vi "strerror.vi"(11 "status_code":u32(ring) items=["APDM_OK"=0, "APDM_INVALID_PARAM"=1, "APDM_MISSED_DATA"=2, "APDM_INITIALIZATION_ERROR"=3, "APDM_NO_MORE_DATA"=4, "APDM_FT_COMMUNICATIONS_ERROR"=5, "APDM_STATUS_ERROR"=6, "APDM_STATUS_UNKNOWN"=7, "APDM_MEMORY_ALLOCATION_ERROR"=8, "APDM_INSUFFICIENT_RESOURCES"=9, "APDM_COMMUNICATIONS_ERROR"=10, "APDM_NOT_ENOUGH_ACCESS_POINTS"=11, "APDM_INVALID_FIRMWARE"=12, "APDM_CANT_RESET_INTO_TARGET_MODE"=13, "APDM_FIRMWARE"=14, "APDM_BOOTLOADER"=15, "APDM_INVALID_CONTEXT_HANDLE"=16, "APDM_CRC16_ERROR"=17, "APDM_DEVICE_RESPONSE_ERROR"=18, "APDM_DEVICE_FIRMWARE_TOO_OLD"=19, "APDM_FILE_ERROR"=20, "APDM_UNSUPPORTED_DEVICE_FIRMWARE_VERSION"=21, "APDM_UNSUPPORTED_DOCKING_STATION_FIRMWARE_VERSION"=22, "APDM_UNSUPPORTED_AP_FIRMWARE_VERSION"=23, "APDM_UNSUPPORTED_CALIBRATION_DATA_VERSION"=24, "APDM_SYNC_LINE_ERROR"=25, "APDM_UNKNOWN_SENSOR_ID_ERROR"=26, "APDM_DEVICE_NOT_FOUND"=27, "APDM_UNSUPPORTED_COMMAND"=28, "APDM_DEVICE_TX_RX_COLLISION_ERROR"=29, "APDM_READ_TIMEOUT_ERROR"=30, "APDM_UNABLE_TO_SYNC_RECORD_HEAD_LIST_ERROR"=31, "APDM_UNKNOWN_CALIBRATION_DATA_STRUCTURE"=32, "APDM_NULL_PARAMETER_ERROR"=33, "APDM_NOT_FOUND"=34, "APDM_UNKNOWN_DEVICE_TYPE"=35, "APDM_NO_CORRELATION_FIFO"=36, "APDM_UNSUPPORTED_DATA_FILE_VERSION"=37, "APDM_CORRUPT_DISK_FIFO"=38, "APDM_DOCK_UNSUPPORTED_HOST_LIBRARY_VERSION"=39, "APDM_AP_UNSUPPORTED_HOST_LIBRARY_VERSION"=40, "APDM_UNEXPECTED_STRUCTURE_VALUE"=41, "APDM_BAD_DATA"=42, "APDM_CORRUPT_CONTEXT"=43, "APDM_AP_READ_TIMEOUT_ERROR"=44, "APDM_MONITOR_READ_TIMEOUT_ERROR"=45, "APDM_DOCK_READ_TIMEOUT_ERROR"=46, "APDM_DEVICE_RESPONSE_ERROR_CRC_ERROR"=47, "APDM_DEVICE_RESPONSE_ERROR_INVALID_COMMAND"=48, "APDM_DEVICE_RESPONSE_ERROR_INVALID_PARAM_SIZE"=49, "APDM_DEVICE_RESPONSE_ERROR_INVALID_PARAM_VALUE"=50, "APDM_DEVICE_RESPONSE_ERROR_ERROR_EXECUTING_COMMAND"=51, "APDM_RECALIBRATION_INSUFFICIENT_DATA"=52, "APDM_RECALIBRATION_BAD_FIT"=53, "APDM_RECALIBRATION_INSUFFICIENT_MOVEMENT"=54, "APDM_FIRMWARE_COMBINATION_ERROR"=55, "APDM_DATA_FROM_UNEXPECTED_MONITOR_ERROR"=56, "APDM_ORIENTATION_ERROR"=57, "APDM_UNABLE_TO_PING_MONITOR_ERROR"=58, "APDM_FIRMWARE_INCOMPATABLE"=59, "APDM_INVALID_MONITOR_CONFIGURATION"=60, "APDM_UNABLE_TO_MATCH_EXPECTED_AP_IDS"=61, "APDM_AP_LIBUSB_ERROR_NO_DEVICE"=62, "APDM_DOCK_LIBUSB_ERROR_NO_DEVICE"=63, "APDM_UNSUPPORTED_AP_HANDLE_VERSION"=64, "APDM_NOT_V1_AP_HANDLE"=65, "APDM_NOT_V2_AP_HANDLE"=66, "APDM_NOT_V1_DOCK_HANDLE"=67, "APDM_NOT_V2_MONITOR_HANDLE"=68, "APDM_HANDLE_VERSION_UNKNOWN"=69, "APDM_CANT_MIX_HARDWARE_VERSIONS"=70, "APDM_CORRELATION_ERROR"=71, "APDM_NOT_ENOUGH_MONITORS"=72, "APDM_NO_FILE_OVERLAP"=73, "APDM_ECHO_SYNC_ERROR"=74, "APDM_AP_NOT_READY_TO_STREAM"=75, "APDM_INTERPOLATION_ERROR"=76, "APDM_ASYNC_MODE_RESPONSE"=77, "APDM_COMMUNICATION_MAGIC_NUMBER_ERROR"=78, "APDM_SENSOR_RESET_DURING_STREAMING"=79, "APDM_HDF_ERROR"=80, "APDM_BUFFER_VALIDATION"=81, "APDM_DECOMPRESSION_ERROR"=82, "APDM_DATA_COMM_CRC_ERROR"=83, "APDM_INCORRECT_NUMBER_OF_APS_CONNECTED"=84, "APDM_LIB_USB_ERROR"=2000, "APDM_LIBUSB_ERROR_IO"=2001, "APDM_LIBUSB_ERROR_INVALID_PARAM"=2002, "APDM_LIBUSB_ERROR_ACCESS"=2003, "APDM_LIBUSB_ERROR_NO_DEVICE"=2004, "APDM_LIBUSB_ERROR_NOT_FOUND"=2005, "APDM_LIBUSB_ERROR_BUSY"=2006, "APDM_LIBUSB_ERROR_TIMEOUT"=2007, "APDM_LIBUSB_ERROR_OVERFLOW"=2008, "APDM_LIBUSB_ERROR_PIPE"=2009, "APDM_LIBUSB_ERROR_INTERRUPTED"=2010, "APDM_LIBUSB_ERROR_NO_MEM"=2011, "APDM_LIBUSB_ERROR_NOT_SUPPORTED"=2012, "APDM_LIBUSB_ERROR_UNKOWN"=2098, "APDM_LIBUSB_ERROR_OTHER"=2099, "APDM_FTDI_COMM_ERROR"=3000]) -> (3 "function return":string)   [LabVIEW 2019, in "apdm.lvlib"]
doc: "APDM_EXPORT const char* apdm_strerror(const enum APDM_Status status_code);"
uses:
  apdm.lvlib
  Lee Lab/CP FES Walking 2018/Code/Working/LabVIEW/apdm.dll
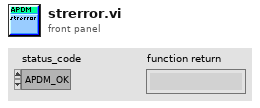
[diagram p1: front panel]
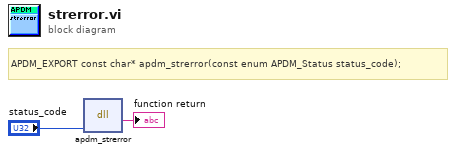
[diagram p0: block diagram]
diagram:
  # "APDM_EXPORT const char* apdm_strerror(const enum APDM_Status status_code);"
  n1 = dll-call lib="C:/Users/jfalesi/Dropbox/Lee Lab/CP FES Walking 2018/Code/Working/LabVIEW/apdm.*" fn="apdm_strerror"("status_code"="status_code") -> (→"function return":string)  [unwired: 4 in, 2 out]
